vi "add_interpolation_results.vi"(8 "error in (no error)":errorcluster, 10 "data array":string[](array[string]), 11 "Analysis in":refnum<class "Analysis.lvclass">) -> (0 "error out":errorcluster, 2 "data array out":string[](array[string]), 3 "Analysis out":refnum<class "Analysis.lvclass">)   [LabVIEW 2015]
doc: "input is the data array from the text file.\nThe VI searches for theinterpolation results and writes the data into the AnalysisObject"
uses:
  MSControl/Classes/Analysis/Analysis.lvclass
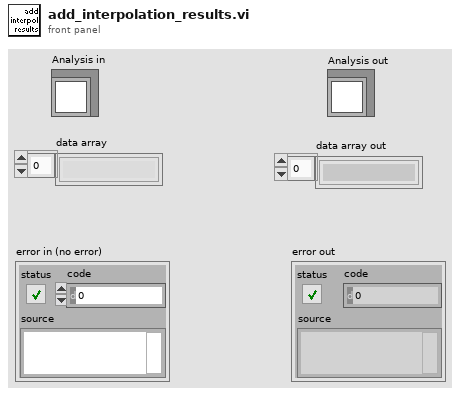
[diagram p1: front panel]
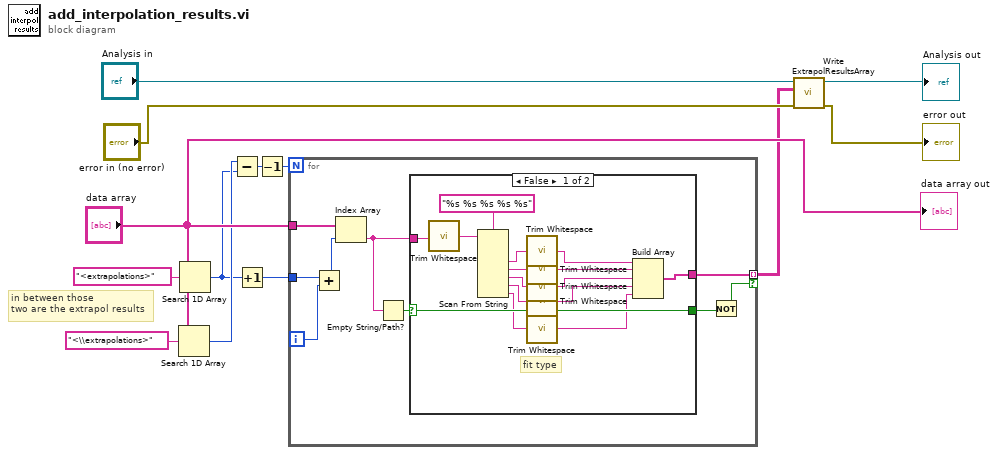
[diagram p0: block diagram]
diagram:
  # "in between those\ntwo are the extrapol results"
  n1 = Search 1D Array(1D array="data array", element="<\\extrapolations>") -> (index of element=w10:i32)  [unwired: 1 in]
  n2 = Search 1D Array(1D array="data array", element="<extrapolations>") -> (index of element=w3:i32)  [unwired: 1 in]
  n3 = Subtract(x=w10, y=w3) -> (x-y=w2:i32)
  n4 = Increment(x=w3) -> (x+1=w4:i32)
  n5 = Decrement(x=w2) -> (x-1=w1:i32)
  n6 = for {
    N: w1 -> [_]
    tunnel: "data array" -> [w22]
    tunnel: w4 -> [w21]
    tunnel: [w18] -> w7 mode=indexing if=w15
    i -> [w20]
    n7 = Add(x=w21, y=w20) -> (x+y=w19:i32)
    n8 = Index Array(array=w22, index=w19) -> (element=w17:string)
    n9 = Empty String/Path?(string/path=w17) -> (empty?=w16:bool)
    n10 = case shown="False" w16 {
      selector: w16 -> [w33 w38]
      tunnel: [w35 _] -> w18
      tunnel: w17 -> [w34 _]
      tunnel: [w33 w38] -> w14
      frame False {
        # "fit type"
        n11 = call <vilib>:"Trim Whitespace.vi"("string"=w34) -> ("trimmed string"=w37:string)  [unwired: 1 in]
        n12 = Scan From String(format string="%s %s %s %s %s", input string=w37) -> (output 1=w32:string, output 2=w31:string, output 3=w30:string, output 4=w29:string, output 5=w24:string)  [unwired: 7 in, 3 out]
        n13 = call <vilib>:"Trim Whitespace.vi"("string"=w32) -> ("trimmed string"=w28:string)  [unwired: 1 in]
        n14 = call <vilib>:"Trim Whitespace.vi"("string"=w31) -> ("trimmed string"=w27:string)  [unwired: 1 in]
        n15 = call <vilib>:"Trim Whitespace.vi"("string"=w30) -> ("trimmed string"=w26:string)  [unwired: 1 in]
        n16 = call <vilib>:"Trim Whitespace.vi"("string"=w29) -> ("trimmed string"=w25:string)  [unwired: 1 in]
        n17 = call <vilib>:"Trim Whitespace.vi"("string"=w24) -> ("trimmed string"=w23:string)  [unwired: 1 in]
        n18 = Build Array(w28, w27, w26, w25, w23) -> (w35:string[])
      }
      frame True {
      }
    }
    n19 = Not(x=w14) -> (.not. x?=w15:bool)
  }
  n20 = call-dynamic "Write ExtrapolResultsArray.vi"("error in (no error)"="error in (no error)", "ExtrapolResultsArray"=w7, "Analysis in"="Analysis in") -> ("error out"=→"error out":errorcluster, "Analysis out"=→"Analysis out":refnum<class "Analysis.lvclass">)  [unwired: 7 in]
  "data array out" <- "data array"
